vi "PH_Sixpack.EmergencyStop.vi"(0 "i ref in":refnum<vi>, 5 "error in":errorcluster) -> (14 "i ref out":refnum<vi>, 18 "Device Error out":errorcluster, 19 "error out":errorcluster)   [LabVIEW 2014, in "PH_Sixpack.lvlib"]
doc: "Stopps all motors at the same time."
uses:
  PH_Sixpack.lvlib
  instr.lib/SixPack/Sixpack - Driver.lvlib
  PH_Stepmotor_BaseClass/PH_Stepmotor_BaseClass.lvlib
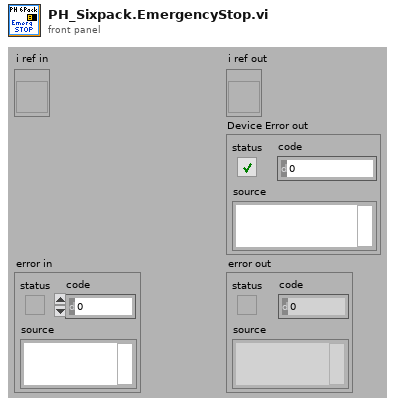
[diagram p1: front panel]
types:
  T1 = cluster{"Motor 0":bool, "Motor 1":bool, "Motor 2":bool, "Motor 3":bool, "Motor 4":bool, "Motor 5":bool}
  T2 = typedef "PH_Sixpack.lvlib/PH_Sixpack.i attribute.ctl" = cluster{"Information":cluster{"SixPack ID(0)":u16, "BaudRate(19200)":u16, "COM Port":enum32{"COM1", "COM2", "COM3", "COM4", "COM5", "COM6", "COM7", "COM8", "COM9"}, "HANDLE":i32}, "Serial Number":dbl, "Firmwareversion":dbl, "Axes":T3[], "Status":T15, "Axis to do a RefSearch":i32, "GUI Refs":cluster{"Information":refnum<vi>, "Serial Number":refnum<vi>, "Firmwareversion":refnum<vi>, "Status":refnum<vi>, "Axis to do a RefSearch":refnum<vi>, "Axes Configuration (Sixpack)":refnum<vi>, "Inputs":refnum<vi>, "PeriodicInterval [ms]":refnum<vi>}, "Constructor finished":bool, "Ignore Error":bool}
  T3 = typedef "PH_Sixpack.lvlib/PH_Sixpack.Axis Cluster.ctl" = cluster{"Config":T4, "To set?":cluster{"VmaxAmax":bool, "I max":bool, "VStartVminDivi":bool, "Ref Search Parameter":bool, "Stopswitch Limits":bool, "Axis Parameter":bool, "I Control":bool}}
  T4 = typedef "PH_Sixpack.lvlib/PH_Sixpack.Axis Configuration.ctl" = cluster{"VmaxAmax":T5, "I max (50%)":T6, "VStartVminDivi":T7, "Ref Search Parameter":T8, "Stopswitch Limits":T9, "Axis Parameter":T10, "I Control":T13}
  T5 = typedef "Sixpack - Driver.lvlib/VmaxAmax.ctl" = cluster{"VMax(511)":u16, "AMax(128)":u16}
  T6 = typedef "Sixpack - Driver.lvlib/PeakCurrent.ctl" = dbl
  T7 = typedef "Sixpack - Driver.lvlib/VStartVmin.ctl" = cluster{"VStart(5)":u16, "Vmin(4)":u16, "Div i (2)":enum8{"0", "1", "2", "3"}}
  T8 = typedef "Sixpack - Driver.lvlib/Ref Search Parameter.ctl" = cluster{"VRefMax(100)":u16, "DebouncingTime (22ms)":u8}
  T9 = typedef "Sixpack - Driver.lvlib/Stopswitch Limits.ctl" = cluster{"MinLeft(0)":u16, "MaxRight(1023)":u16}
  T10 = typedef "Sixpack - Driver.lvlib/Motor Parameter.ctl" = cluster{"Poslimit (6400)":u32, "P5 Bits":T11, "P6 Bits":T12}
  T11 = typedef "Sixpack - Driver.lvlib/MotorParameter_P5.ctl" = cluster{"MT_PI":bool, "MT_ROTARY":bool, "MT_AUTONULLCMD":bool, "MT_TESTNULL":bool, "MT_NULLLEFT":bool, "MT_NULLCENTRE":bool, "MT_STOPNULL":bool, "MT_FILTERSWITCH":bool}
  T12 = typedef "Sixpack - Driver.lvlib/MotorParameter_P6.ctl" = cluster{"MT_OPTIMIZEWAY":bool, "MT_FASTREF":bool, "MT_MECHREF":bool, "MT_DELAYTESTNULL":bool, "MT_STOPSOFT":bool, "MT_STOPNOREF":bool, "MT_NULLPOSITIVE":bool, "MUT_STOPFULSTEPS":bool}
  T13 = typedef "Sixpack - Driver.lvlib/Current Control.ctl" = cluster{"PowerDownDelay (500)":u16, "PowerDown (0%)":T14, "Standing (50%)":T14, "Running (75%)":T14, "Accelerating (100%)":T14}
  T14 = typedef "Sixpack - Driver.lvlib/Current.ctl" = enum8{"100%", "75%", "50%", "38%", "25%", "19%", "13%", "9%", "0%"}
  T15 = typedef "PH_Sixpack.lvlib/PH_Sixpack.Status.ctl" = enum32{"None", "Init", "Configure", "configured", "Close", "closed"}
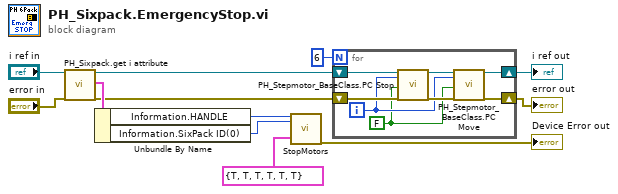
[diagram p0: block diagram]
diagram:
  n1 = call "PH_Sixpack.get i attribute.vi"("i ref in"="i ref in", "error in (no error)"="error in") -> ("i ref out"=w8:refnum<vi>, "i attribute"=w10:T2, "error out"=w7:errorcluster)  [unwired: 15 in]
  n2 = Unbundle By Name(w10) -> ("Information.HANDLE"=w9:i32, "Information.SixPack ID(0)"=w1:u16)
  n3 = call "StopMotors.vi"("handle in"=w9, "UnitAddress(0)"=w1, "Motors"=T1 {"Motor 0"=TRUE, "Motor 1"=TRUE, "Motor 2"=TRUE, "Motor 3"=TRUE, "Motor 4"=TRUE, "Motor 5"=TRUE} ("P0 = Mask for deceleration")) -> ("error out"=→"Device Error out":errorcluster)  [unwired: 15 in, 1 out]
  n4 = for {
    N: 6 -> [_]
    shift-right: [w15] -> w12
    shift-left: w8 -> [w20]
    shift-right: [w17] -> w11
    shift-left: w7 -> [w19]
    i -> [w14]
    w13 = FALSE ("Stop")
    n5 = call "PH_Stepmotor_BaseClass.PC Stop.vi"("i ref in"=w20, "axis"=w14, "Stop"=w13, "error in (no error)"=w19) -> ("i ref out"=w16:refnum<vi>, "error out"=w18:errorcluster)  [unwired: 14 in]
    n6 = call "PH_Stepmotor_BaseClass.PC Move.vi"("i ref in"=w16, "axis"=w14, "Move"=w13, "error in (no error)"=w18) -> ("i ref out"=w15:refnum<vi>, "error out"=w17:errorcluster)  [unwired: 14 in]
  }
  "error out" <- w11
  "i ref out" <- w12
